vi "connect.vi"(8 "error in (no error)":errorcluster, 11 "TEST in":refnum<class "TEST.lvclass">) -> (0 "error out":errorcluster, 3 "TEST out":refnum<class "TEST.lvclass">)   [LabVIEW 2019, in "TEST.lvclass"]
uses:
  TEST.lvclass
  D:/my_projects/projects/Algorithms/Labview/19/Modbus/MB_TCP2/MB_TCP.lvclass
  MB_TCP.lvclass/MB_TCP.ctl
  NI_modbus_upd/TCP/TCP.lvclass/TCP.ctl
  NI_modbus_upd/TCP/TCP.lvclass
  MB_TCP.lvclass
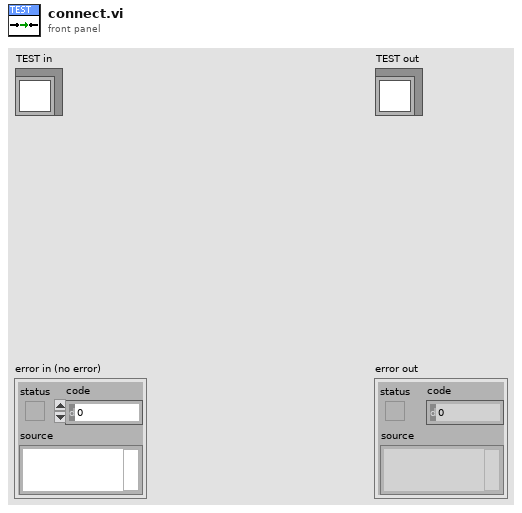
[diagram p1: front panel]
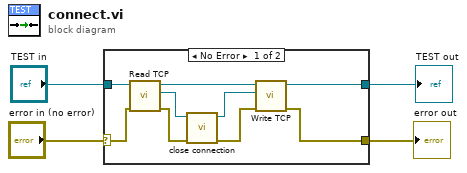
[diagram p0: block diagram]
diagram:
  n1 = case shown="No Error" "error in (no error)" {
    selector: "error in (no error)" -> [w11 w14]
    tunnel: [w6 w14] -> w1
    tunnel: [w5 w15] -> w2
    tunnel: "TEST in" -> [w13 w15]
    frame No Error {
      n2 = call "Read TCP.vi"("error in (no error)"=w11, "MB_TCP in"=w13) -> ("error out"=w10:errorcluster, "TCP"=w12:refnum<class "TCP.lvclass">, "MB_TCP out"=w9:refnum<class "TEST.lvclass">)  [unwired: 7 in]
      n3 = call "close connection.vi"("error in (no error)"=w10, "TCP in"=w12) -> ("error out"=w7:errorcluster, "TCP out"=w8:refnum<class "TCP.lvclass">)  [unwired: 8 in]
      n4 = call "Write TCP.vi"("error in (no error)"=w7, "TCP"=w8, "MB_TCP in"=w9) -> ("error out"=w6:errorcluster, "MB_TCP out"=w5:refnum<class "TEST.lvclass">)  [unwired: 7 in]
    }
    frame Error {
    }
  }
  "error out" <- w1
  "TEST out" <- w2
